vi "BestSolution&ItsIndex.vi"(11 "Population":T1[](array[typedef])) -> (2 "Best Solution In the Population":T1, 3 "Best Solution Index for Replace":i32)   [LabVIEW 2013, in "GA.lvclass"]
uses:
  GA.lvclass
  Controls/Solution_GA.ctl
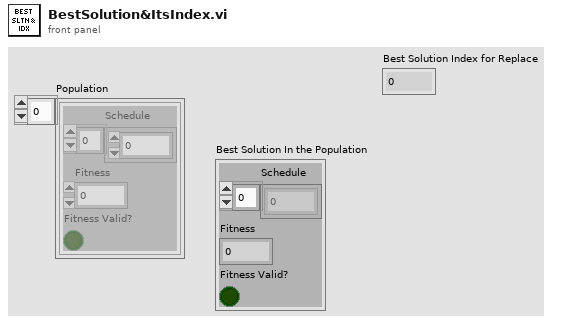
[diagram p1: front panel]
types:
  T1 = typedef "Solution_GA.ctl" = cluster{"Schedule":u16[], "Fitness":u16, "Fitness Valid?":bool}
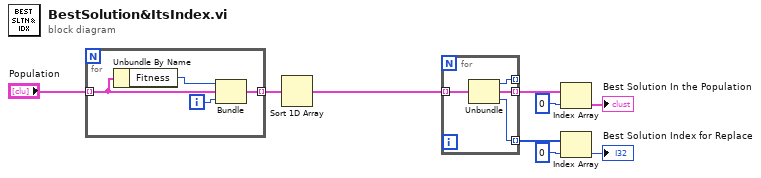
[diagram p0: block diagram]
diagram:
  n1 = for {
    tunnel: "Population" -> [w12] mode=indexing
    tunnel: [w11] -> w7 mode=indexing
    i -> [w10]
    n2 = Unbundle By Name(w12) -> ("Fitness"=w13:u16)
    n3 = Bundle("Fitness"=w13, "Solution"=w12, w10) -> (w11:cluster{"Fitness":u16, "Solution":T1, i32})  [unwired: 1 in]
  }
  n4 = Sort 1D Array(array=w7) -> (sorted array=w6:cluster{"Fitness":u16, "Solution":T1, i32}[])
  n5 = for {
    tunnel: w6 -> [w17] mode=indexing
    tunnel: [w16] -> w5 mode=indexing
    tunnel: [w15] -> _ mode=indexing
    tunnel: [w14] -> w3 mode=indexing
    n6 = Unbundle(w17) -> ("Fitness"=w15:u16, "Solution"=w16:T1, w14:i32)
  }
  n7 = Index Array(array=w5, index=0) -> (element=→"Best Solution In the Population":T1)
  n8 = Index Array(array=w3, index=0) -> (element=→"Best Solution Index for Replace":i32)
